vi "Telnet_Receive.vi"(8 "Error In":errorcluster caption="Entrée d'erreur", 9 "timeout ms (100)":i32=100, 10 "Console in":string, 11 "telnet connection in":T1) -> (0 "Error Out":errorcluster caption="Sortie d'erreur", 1 "NewData":string, 2 "Console out":string, 3 "telnet connection out":T1, 5 "NewData":bool)   [LabVIEW 2013]
uses:
  <vilib>/addons/internet/telnet/telnet.llb/Telnet Session.ctl
  <vilib>/addons/internet/NI_InternetTK_Core_VIs.lvlib
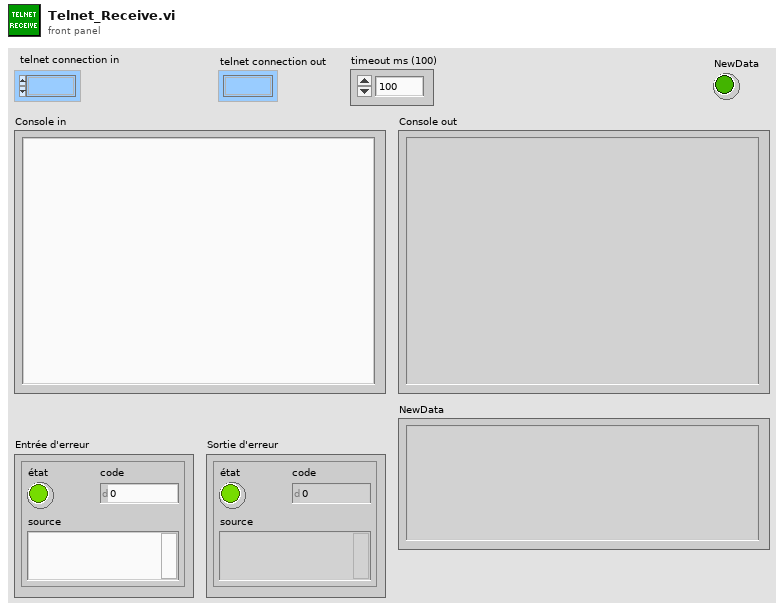
[diagram p1: front panel]
types:
  T1 = typedef "Telnet Session.ctl" = refnum<k1>
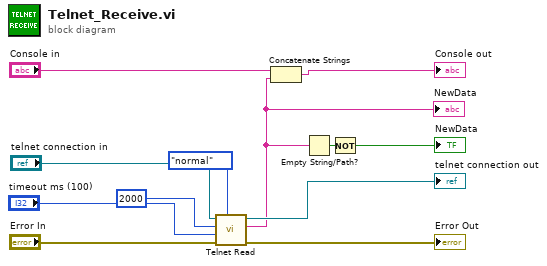
[diagram p0: block diagram]
diagram:
  n1 = call <vilib>:"Telnet Read.vi"("read mode (normal)"=enum16{"normal", "line", "buffered"}."normal", "error in (no error)"="Error In", "timeout ms (25000)"="timeout ms (100)", "bytes to read"=2000, "telnet connection"="telnet connection in") -> ("error out"=→"Error Out":errorcluster, "data out"=w2:string, "telnet connection out"=→"telnet connection out":T1)  [unwired: 2 in]
  "NewData" <- w2
  n2 = Concatenate Strings("Console in", w2) -> (→"Console out":string)
  n3 = Empty String/Path?(string/path=w2) -> (empty?=w4:bool)
  n4 = Not(x=w4) -> (.not. x?=→"NewData":bool)
